vi "Open System Definition.vi"(8 "error in (no error)":errorcluster, 11 "System Definition File":path) -> (0 "error out":errorcluster, 1 "Target Refnum":refnum<k24>, 2 "Root Refnum":refnum<k24>, 3 "System Definition Refnum":refnum<k24>)   [LabVIEW 2019, in "NI-SWITCH Examples.lvlib"]
uses:
  NI-SWITCH Examples.lvlib
  NationalInstruments.VeriStand.SystemDefinitionAPI
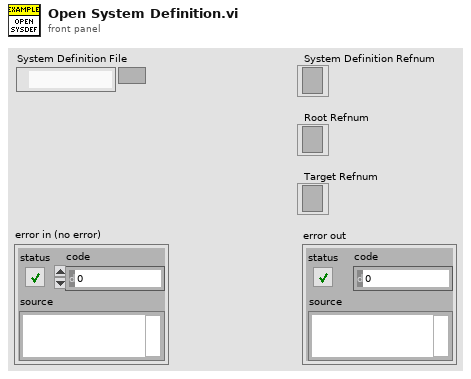
[diagram p1: front panel]
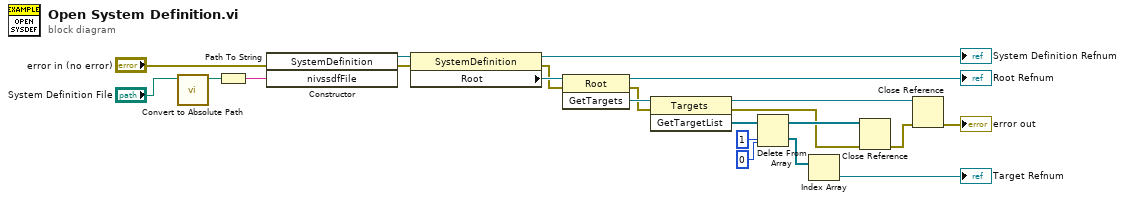
[diagram p0: block diagram]
diagram:
  n1 = call "Convert to Absolute Path.vi"("System Definition File"="System Definition File") -> ("Absolute Path"=w1:path)  [unwired: 10 in]
  n2 = Path To String(path=w1) -> (string=w3:string)
  n3 = constructor class="SystemDefinition"(error in="error in (no error)", "nivssdfFile"=w3) -> (reference out=w6:refnum<k24>, error out=w5:errorcluster)  [unwired: 2 in, 2 out]
  n4 = property class="SystemDefinition"(reference=w6, error in=w5) -> (reference out=→"System Definition Refnum":refnum<k24>, error out=w7:errorcluster, "Root"=w8:refnum<k24>)
  n5 = invoke class="Root" method="GetTargets"(reference=w8, error in=w7) -> (reference out=→"Root Refnum":refnum<k24>, error out=w9:errorcluster, "GetTargets"=w10:refnum<k24>)  [unwired: 1 in]
  n6 = invoke class="Targets" method="GetTargetList"(reference=w10, error in=w9) -> (reference out=w17:refnum<k24>, error out=w14:errorcluster, "GetTargetList"=w11:refnum<k24>[])  [unwired: 1 in]
  n7 = Delete From Array(array=w11, length=1, index=0) -> (deleted portion=w18:refnum<k24>[], array with subset deleted=w15:refnum<k24>[])
  n8 = Index Array(array=w18) -> (element=→"Target Refnum":refnum<k24>)  [unwired: 1 in]
  n9 = Close Reference(reference=w15, error in (no error)=w14) -> (error out=w16:errorcluster)
  n10 = Close Reference(reference=w17, error in (no error)=w16) -> (error out=→"error out":errorcluster)
